vi "mag_resp.vi"() -> ()   [LabVIEW 2010]
uses:
  <vilib>/addons/Digital Filter Design/Analysis.llb/DFD Plot Freq Response (Linear-Spaced).vi
  <vilib>/addons/Digital Filter Design/NI_DigFilterLicensed.lvlib
  <vilib>/Analysis/NI_AALBase.lvlib
panel:
  in  "order":i32=2
  in  "# of taps":i32=501
  in  "high freq":dbl=500000.0 format="%#_3p"
  in  "stop freq":dbl=300000.0 format="%#_3p"
  out "magnitude response":cluster{"f0":dbl, "df":dbl, "values":dbl[]}[](graph)
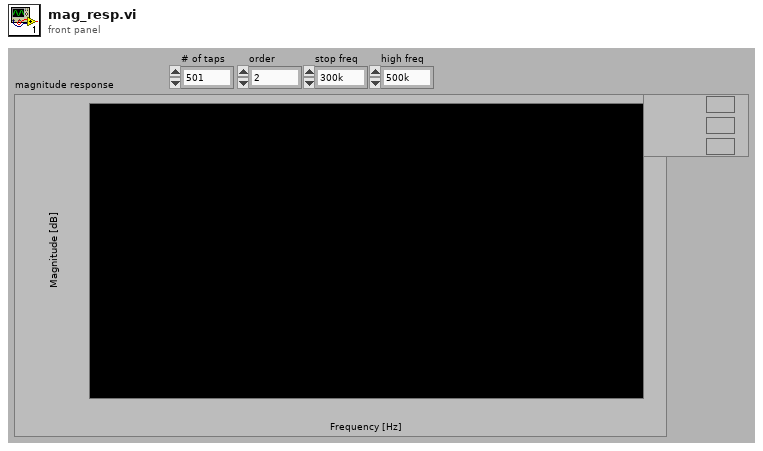
[diagram p1: front panel]
types:
  T1 = enum16{"Lowpass", "Highpass", "Bandpass", "Bandstop"}
  T2 = cluster{"Amplitude":dbl, "DC":dbl, "stop freq":dbl, "Weight":dbl}
  T3 = cluster{"Amplitude":dbl, "high freq":dbl, dbl, "Weight":dbl}
  T4 = cluster{"Amplitude":dbl, "high freq":dbl, "stop freq":dbl, "Weight":dbl}[]
  T5 = typedef "NI_DigFilterLicensed.lvlib/DFD Filter Obj.ctl" = cluster{"mSRate_Fs":dbl, "mSRate_Version":string, "mSRate_Comments":string, "mSRate_OrgCoef":T6, "mSRate_CurCoef":T6, "mSRate_Quantized?":bool, "mSRate_QCoef":T6, "mSRate_QSettings":T8[], "mSRate_Order":i32, "mSRate_Scaling":cluster{"mSRate_ScaleByPowerOf2?":bool, "mSRate_ScaleType":T10}}
  T6 = typedef "NI_DigFilterLicensed.lvlib/DFD Filter Coef.ctl" = cluster{"type":T7, "gain":dbl, "coef a (k)":dbl[], "coef b (v)":dbl[]}
  T7 = typedef "NI_DigFilterLicensed.lvlib/DFD Filter Structure Type Selector.ctl" = enum16{"Undefined", "FIR Direct Form", "FIR Direct Form Transposed", "FIR Symmetric", "FIR Antisymmetric", "IIR Direct Form I", "IIR Direct Form I Transposed", "IIR Direct Form II", "IIR Direct Form II Transposed", "IIR Cascaded Second Order Sections Form I", "IIR Cascaded Second Order Sections Form I Transposed", "IIR Cascaded Second Order Sections Form II", "IIR Cascaded Second Order Sections Form II Transposed", "Lattice Allpass (basic sections)", "Lattice Allpass (one multiplier sections)", "Lattice Allpass (normalized sections)", "Lattice AR (basic sections)", "Lattice AR (one multiplier sections)", "Lattice AR (normalized sections)", "Lattice MA (minimum phase)", "Lattice MA (maximum phase)", "Lattice ARMA (basic sections)", "Lattice ARMA (one multiplier sections)", "Lattice ARMA (normalized sections)"}
  T8 = typedef "NI_DigFilterLicensed.lvlib/dfd_Internal Quantization Settings.ctl" = cluster{"source":T9, "wl":i16, "iwl":i16, "overflow mode":enum16{"Saturation", "Wrap"}, "rounding mode":enum16{"Nearest", "Truncation"}, "signed?":bool}
  T9 = typedef "NI_DigFilterLicensed.lvlib/dfd_Internal Quantization Srcs.ctl" = u16
  T10 = typedef "NI_DigFilterLicensed.lvlib/DFD Coef Norm Type.ctl" = enum16{"No Norm", "Time Domain 1-Norm", "Time Domain 2-Norm", "Time Domain Inf-Norm"}
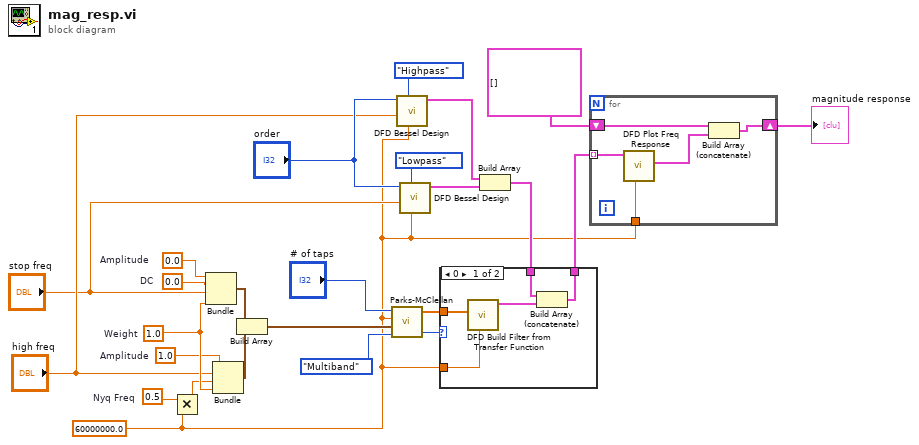
[diagram p0: block diagram]
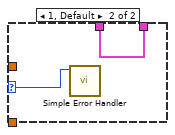
[diagram p2: hidden frame]
diagram:
  w14 = 1.0  # Weight
  w9 = 0.5  # Nyq Freq
  w13 = 1.0  # Amplitude
  w16 = 0.0  # DC
  w15 = 0.0  # Amplitude
  w1 = 60000000.0 ("fs [Hz]")
  n1 = Multiply(x=w9, y=w1) -> (x*y=w10:dbl)
  n2 = Bundle("Amplitude"=w15, "DC"=w16, "stop freq"="stop freq", "Weight"=w14) -> (w11:T2)  [unwired: 1 in]
  n3 = Bundle("Amplitude"=w13, "high freq"="high freq", w10, "Weight"=w14) -> (w12:T3)  [unwired: 1 in]
  n4 = Build Array(w11, w12) -> (w8:T4)
  n5 = call <vilib>:"Parks-McClellan.vi"("filter type"=enum32{"Multiband", "Differentiator", "Hilbert"}."Multiband", "Band Parameters"=w8, "sampling freq: fs"=w1, "# of taps"="# of taps") -> ("error"=w5:i32, "h"=w7:dbl[])  [unwired: 1 out]
  n6 = call <vilib>:"DFD Bessel Design.vi"("fs [Hz]"=w1, "filter type"=T1."Highpass", "low cutoff freq [Hz]"="high freq", "order"="order") -> ("filter out"=w22:T5)  [unwired: 6 in, 1 out]
  n7 = call <vilib>:"DFD Bessel Design.vi"("fs [Hz]"=w1, "filter type"=T1."Lowpass", "low cutoff freq [Hz]"="stop freq", "order"="order") -> ("filter out"=w19:T5)  [unwired: 6 in, 1 out]
  n8 = Build Array(w22, w19) -> (w6:T5[])
  n9 = case shown="0" w5 {
    selector: w5 -> [_ w32]
    tunnel: w7 -> [w30 _]
    tunnel: w6 -> [w29 w31]
    tunnel: [w27 w31] -> w4
    tunnel: w1 -> [w26 _]
    frame 0 {
      n10 = call <vilib>:"DFD Build Filter from Transfer Function.vi"("fs [Hz]"=w26, "numerator"=w30) -> ("filter out"=w28:T5)  [unwired: 2 in, 7 out]
      n11 = Build Array (concatenate)(w29, w28) -> (w27:T5[])
    }
    frame 1, Default {
      n12 = call <vilib>:"Simple Error Handler.vi"("error code (no error:0)"=w32) -> ()  [unwired: 4 in, 5 out]
    }
  }
  n13 = for {
    tunnel: w1 -> [w37]
    tunnel: w4 -> [w36] mode=indexing
    shift-right: [w34] -> w21
    shift-left: cluster{"f0":dbl, "df":dbl, "values":dbl[]}[] [] -> [w33]
    n14 = call-poly <vilib>:"DFD Plot Freq Response.vi"("fs [Hz]"=w37, "filter in"=w36) -> ("magnitude response"=w35:cluster{"f0":dbl, "df":dbl, "values":dbl[]}[])  [unwired: 6 in, 3 out]
    n15 = Build Array (concatenate)(w33, w35) -> (w34:cluster{"f0":dbl, "df":dbl, "values":dbl[]}[])
  }
  "magnitude response" <- w21
